vi "Main v0.97.vi"() -> ()   [LabVIEW 2017]
doc: "v0.85:\n- Counts for rejects and total\n\nv0.5:\n\n- Added Reject to Manual Mode\n- Send reject pallet cluster during manual mode\n- Run continuous manual happens only when no error has occured"
uses:
  Controls/Main Tabs v0.1.ctl
  Controls/Auto.ctl
  RT/Controls/Auto Delays.ctl
  RT/Controls/Auto Times.ctl
  Controls/UI Data.ctl
  support/Controls/Auto Stats.ctl
  support/Message Queue/Enqueue Message (Single).vi
  GV/Maintenance GV.vi
  <vilib>/Utility/error.llb/Error Cluster From Error Code.vi
  <vilib>/ErrorRing/Error Ring.xnode
  support/Message Queue/Message Queue.lvlib
  support/User Event - Stop/User Event - Stop.lvlib
panel:
  out "Shutdown?":bool
  out "Boolean 8":bool
  out "Boolean 7":bool
  out "Boolean 6":bool
  out "Boolean 5":bool
  out "Boolean 4":bool
  out "Boolean 3":bool
  out "Boolean 2":bool
  out "Boolean":bool
  in  "Reject Pallets":T1
  out "Date-Time":string caption="Dip-Tube Assembly Automation (HMI) v0.9"
  out "Main Tab":T2
  in  "Autocycle":T3
  in  "Manual":bool
  in  "Parameters":bool
  in  "Maintenance":bool
  in  "BF Para":cluster{"Delay 1":u32, "Delay 2":u32}={"Delay 1"=1000, "Delay 2"=1000}
  in  "Reject Para":cluster{"Delay":u32}={"Delay"=400}
  in  "Meas. Para":T4={"Delay"=500.0, "Mean Length"=188.9, "Tolerance"=1.0}
  in  "PF Para":cluster{"Delay":u32, "Timeout":u32}={"Delay"=1000, "Timeout"=1000}
  in  "Tube Feeder Para":T5={"Delay"=400, "Delay 2"=250, "Max Attempts"=250}
  in  "Cutting Para":T6={"Delay"=400, "Delay 2"=250, "Delay 3"=250}
  in  "Agitator Para":cluster{"Delay":u32, "Timeout":u32}={"Delay"=400, "Timeout"=250}
  in  "Insertion Para":cluster{"Delay 1":u32, "Delay 2":u32}={"Delay 1"=1000, "Delay 2"=1000}
  in  "Save Para":bool
  in  "Home Para":bool
  out "OEE":dbl format="%#.1f"
  out "QUA":dbl=100.0 min=0.0 max=100.0 step=0.1
  in  "Ideal Time":dbl=2.0 min=0.0 max=100.0 step=0.1
  in  "AVL":dbl=100.0 min=0.0 max=100.0 step=0.1
  out "Rejects 2":u32
  in  "Reset MCount":bool
  in  "Enable BF?":bool
  in  "Enable Agitate?":bool
  in  "Enable Reject?":bool
  in  "Toggle Motor":bool
  in  "Continuous?":bool
  in  "Enable Measure?":bool
  in  "Enable Index?":bool
  in  "Enable PF?":bool
  in  "Auto Para":T7={"Agitator Delays"=[400, 250], "TF Delays"=[700, 800, 2], "Insertion Delays"=[100, 500], "Cutting Delays"=[300, 300, 100], "PF Delays"=[250, 30000], "Measur. Delays"=[500.0, 188.9, 1.0], "Reject Delays"=[500], "BF Delays"=[1000, 1000]}
  in  "Enable Cutting?":bool
  in  "Enable Insertion?":bool
  in  "Run Manual":bool
  in  "Enable TF?":bool
  in  "Home Manual":bool
  out "Status 2":T9
  out "Measurements":T10 {"Height 1" format="%#.2f"; "Height 2" format="%#.2f"; "Height 3" format="%#.2f"; "Height 4" format="%#.2f"}
  out "Output Count":u32 caption="Output\nCount"
  out "PRF":dbl=100.0 min=0.0 max=100.0 step=0.1
  out "Statuses":string[][](table)
  in  "All IO":bool
  in  "Stats":bool
  in  "Home AC":bool
  out "Status":string
  out "Count":u32 format="%06.0f"
  out "Cycle Time":dbl format="%0.2f"
  out "Rejects":u32 format="%06.0f"
  out "Output Chart":T11(graph)
  out "Reject Count":u32
  out "Total Count":u32
  out "Total Time":dbl caption="Total Effective Cycle Time (s)" format="%#.3f"
  out "Time Chart":T12(graph)
  out "OEE Chart":cluster{"1":dbl, "2":dbl, "3":dbl, "4":dbl}(graph)
  out "Measurement Chart":cluster{"1":dbl, "2":dbl, "3":dbl, "4":dbl}(graph)
  out "Timestamp":string caption="Date & Timestamp"
  out "Latest Measure.":T13 caption="Latest Measurements" {"Length 1 (mm)" format="%#.2f"}
  out "Auto Times":T8
  in  "Back Stats":bool
  out "OEE 2":T14 caption="Latest Measurements" {"AVL" format="%#.1f"; "PRF" format="%#.1f"; "QUA" format="%#.1f"; "OEE" format="%#.1f"}
  out "IAS 4":dbl format="%#.3f"
  out "IAS 3":dbl format="%#.3f"
  out "IAS 2":dbl format="%#.3f"
  out "IAS 1":dbl format="%#.3f"
  out "DI 1":T15
  out "DI 2":T16
  out "DO 1":T17
  in  "Back IO":bool
  in  "Exit":bool
  in  "Shutdown":bool
  # "HARMONY VISION DIP-TUBE ASSEMBLY AUTOMATION"
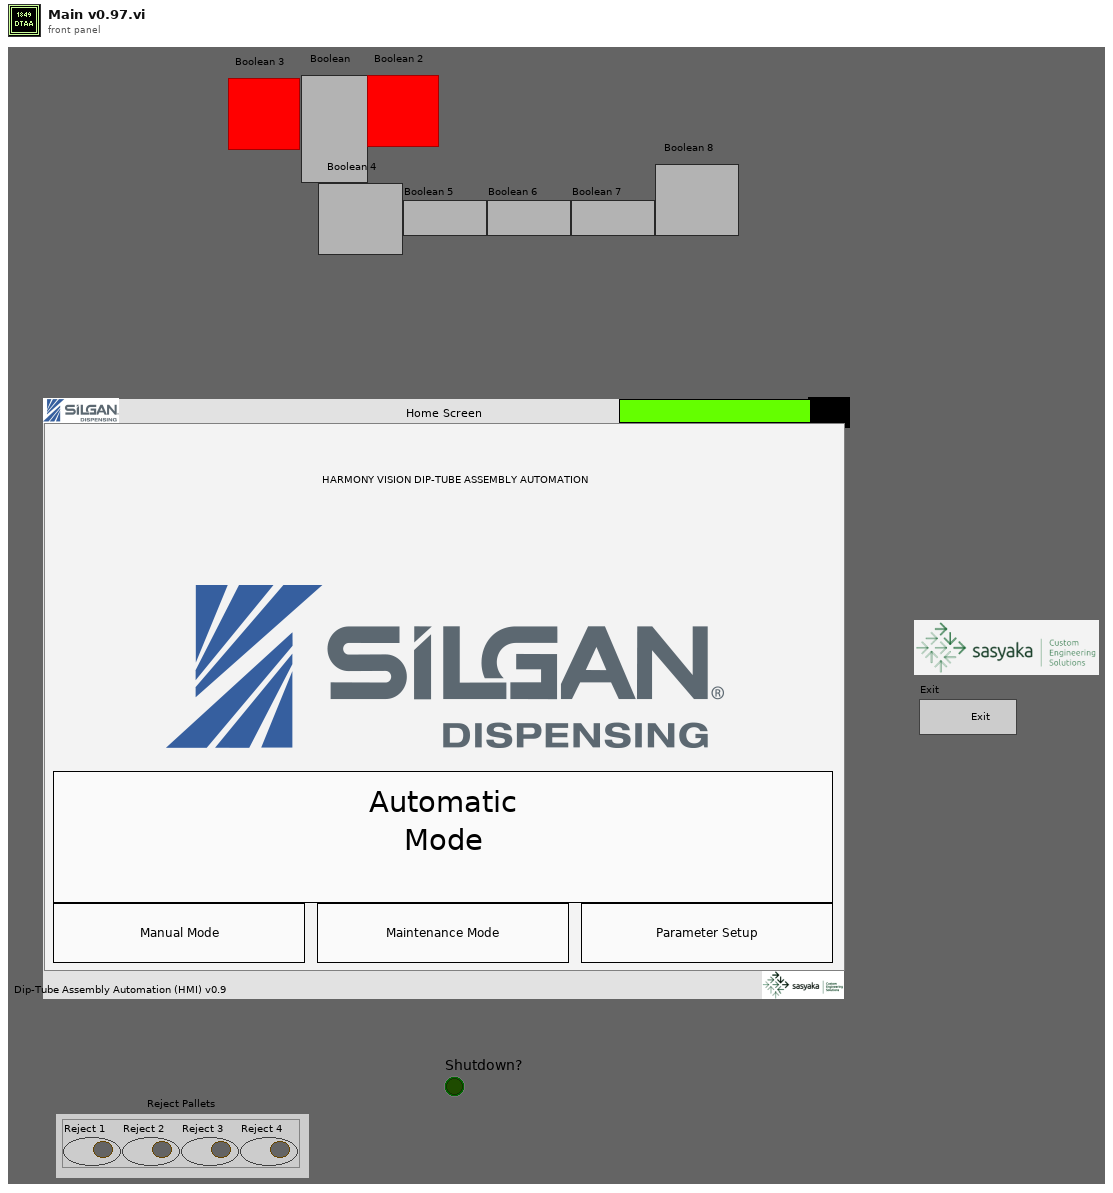
[diagram p1: front panel]
types:
  T1 = cluster{"Reject 1":bool, "Reject 2":bool, "Reject 3":bool, "Reject 4":bool}
  T2 = typedef "Main Tabs v0.1.ctl" = enum32{"Home Screen", "Parameter Setup", "Manual Mode", "Autocycle", "Autocycle Statistics", "Autocycle IOs"}
  T3 = typedef "Auto.ctl" = bool
  T4 = cluster{"Delay":dbl, "Mean Length":dbl, "Tolerance":dbl}
  T5 = cluster{"Delay":u32, "Delay 2":u32, "Max Attempts":u32}
  T6 = cluster{"Delay":u32, "Delay 2":u32, "Delay 3":u32}
  T7 = typedef "Auto Delays.ctl" = cluster{"Agitator Delays":u32[], "TF Delays":u32[], "Insertion Delays":u32[], "Cutting Delays":u32[], "PF Delays":u32[], "Measur. Delays":dbl[], "Reject Delays":u32[], "BF Delays":u32[]}
  T8 = typedef "Auto Times.ctl" = cluster{"Index Time":u32, "TF Time":u32, "Insertion Time":u32, "Cutting Time":u32, "PF Time":u32, "Meas. Time":u32, "Reject Time":u32}
  T9 = cluster{"Auto Times":T8, "error out":errorcluster}
  T10 = cluster{"Height 1":dbl, "Height 2":dbl, "Height 3":dbl, "Height 4":dbl}
  T11 = cluster{"OutputCount":u32, "Numeric Control":u32}
  T12 = cluster{"Index":dbl, "TF":dbl, "Insert":dbl, "Cutting":dbl, "PF":dbl, "Measure.":dbl, "Reject":dbl}
  T13 = cluster{"Length 1 (mm)":dbl, "Pallet 2 (mm)":dbl, "Pallet 3 (mm)":dbl, "Pallet 4 (mm)":dbl}
  T14 = cluster{"AVL":dbl, "PRF":dbl, "QUA":dbl, "OEE":dbl}
  T15 = cluster{"Machine_ON":bool, "E_stop ":bool, "SW_Pressure":bool, "SW_Start ":bool, "SW_Reset":bool, "SW_Stop":bool, "SW_Door":bool, "RS_Index_Rotary_CW":bool, "RS_Index_Rotary_CCW":bool, "RS_Index_Stopper _Rear":bool, "RS_Index_Output_Separator_Rear":bool, "PES_Index_Pallet_Sensor":bool, "PES_Index_Output_Part Sensor":bool, "ICS_BF_Low_Level_1":bool, "ICS_BF_Low_Level_2":bool, "ICS_BF_Pump_CNVR_Full_1":bool, "ICS_BF_Pump_CNVR_Full_2":bool, "ICS_BF_Pump_CNVR_Full_3":bool, "ICS_BF_Pump_CNVR_Full_4":bool, "PES_PC_Pump Presence_1":bool, "PES_PC_Pump Presence_2":bool, "PES_PC_Pump Presence_3":bool, "PES_PC_Pump Presence_4":bool, "RS_PC_Gating_Front":bool, "PES_Pump_Interference":bool, "PES_TF_Low_Level":bool, "PES_Tube Presence_1":bool, "PES_Tube Presence_2":bool, "PES_Tube Presence_3":bool, "PES_Tube Presence_4":bool, "DI1.30":bool, "DI1.31":bool}
  T16 = cluster{"RS_Agitatator_1_Rear ":bool, "RS_Agitatator_2_Rear ":bool, "RS_TF_Gating CYL_Rear":bool, "RS_Insertion_1_Rear":bool, "RS_Insertion_1_Front":bool, "RS_Insertion _2_Rear":bool, "RS_Insertion _2_Front":bool, "RS_Insertion _3_Rear":bool, "RS_Insertion _3_Front":bool, "RS_Insertion _4_Rear":bool, "RS_Insertion _4_Front":bool, "RS_Insertion_Clamp_Rear":bool, "RS_Cutting_Rear":bool, "RS_Cutting_Clamp _Rear":bool, "RS_Measurement_1_Rear":bool, "RS_Measurement_2_Rear":bool, "RS_Measurement_3_Rear":bool, "RS_Measurement_4_Rear":bool, "DI2.18":bool, "RS_Rejection_1_Rear":bool, "RS_Rejection_2_Rear":bool, "RS_Rejection_3_Rear":bool, "RS_Rejection_4_Rear":bool, "DI2.23":bool, "DI2.24":bool, "DI2.25":bool, "DI2.26":bool, "DI2.27":bool, "DI2.28":bool, "DI2.29":bool, "DI2.30":bool, "DI2.31":bool}
  T17 = cluster{"TL_Red":bool, "TL_Orange":bool, "TL_Green":bool, "TL_Buzzer":bool, "SOL_Index_Rotary_CW":bool, "SOL_Index_Rotary_CCW":bool, "SOL_Index_Stopper_Rear":bool, "SOL_OutputSeparator_Rear":bool, "Bowl  Feeder_ ON 1":bool, "Pump_CNVR_Motor _ON":bool, "SOL_PC_Gating_CYL_Rear":bool, "SOL_Tube_Feed_Agitatator":bool, "SOL_Tube_Feed_Gating_CYL":bool, "SOL_Insertion _CYL":bool, "SOL_Insertion_Clamp_CYL":bool, "SOL_Cutting_CYL":bool, "SOL_Cutting_Clamp_CYL":bool, "SOL_Insertion_Air_Nozzle":bool, "SOL_Measurement_CYL":bool, "DO1.19":bool, "SOL_Rejection CYL_1":bool, "SOL_Rejection CYL_2":bool, "SOL_Rejection CYL_3":bool, "SOL_Rejection CYL_4":bool, "Bowl  Feeder_ ON 2":bool, "SOL_BF_BlowerON":bool, "SOL_BF1_Track1":bool, "SOL_BF1_Track2":bool, "SOL_BF2_Track1":bool, "SOL_BF2_Track2":bool, "DO1.30":bool, "DO1.31":bool}
  T18 = typedef "UI Data.ctl" = cluster{"Main Tab":refnum<vi>}
  T19 = typedef "Message Queue.lvlib/All Message Queues.ctl" = cluster{"UI":refnum<queue>}
  T20 = enum8{"Enabled", "Disabled", "Disabled and Grayed Out"}
  T21 = cluster{"Array":string[][], "Machine Status":string}
  T22 = typedef "Auto Stats.ctl" = cluster{"Time":timestamp, "OEE":cluster{"AVL":dbl, "PRF":dbl, "QUA":dbl, "OEE":dbl}, "Auto Times":T8, "Counts out":cluster{"OutputCount":u32, "RejectCount":u32}, "Measurements":cluster{"1":dbl, "2":dbl, "3":dbl, "4":dbl}, "Outputs":cluster{"OutputCount":u32, "Numeric Control":u32}}
  T23 = cluster{"Auto Times":T8, "Results":cluster{"Measurements":cluster{"1":dbl, "2":dbl, "3":dbl, "4":dbl}, "Reject Pallets":cluster{"Reject 1":bool, "Reject 2":bool, "Reject 3":bool, "Reject 4":bool}}, "OutputCount":u32, "error out":errorcluster}
  T24 = enum8{"Information", "Error", "Successful", "Tips"}
  T25 = cluster{"Agitator Delays[0]":u32, "Agitator Delays[1]":u32}
  T26 = cluster{"TF Delays[0]":u32, "TF Delays[1]":u32, "TF Delays[2]":u32}
  T27 = cluster{"Insertion Delays[0]":u32, "Insertion Delays[1]":u32}
  T28 = cluster{"Cutting Delays[0]":u32, "Cutting Delays[1]":u32, "Cutting Delays[2]":u32}
  T29 = cluster{"Measur. Delays[0]":dbl, "Measur. Delays[1]":dbl, "Measur. Delays[2]":dbl}
  T30 = typedef "All Inputs.ctl" = cluster{"DI 1":cluster{"Machine_ON":bool, "E_stop ":bool, "SW_Pressure":bool, "SW_Start ":bool, "SW_Reset":bool, "SW_Stop":bool, "SW_Door":bool, "RS_Index_Rotary_CW":bool, "RS_Index_Rotary_CCW":bool, "RS_Index_Stopper _Rear":bool, "RS_Index_Output_Separator_Rear":bool, "PES_Index_Pallet_Sensor":bool, "PES_Index_Output_Part Sensor":bool, "ICS_BF_Low_Level_1":bool, "ICS_BF_Low_Level_2":bool, "ICS_BF_Pump_CNVR_Full_1":bool, "ICS_BF_Pump_CNVR_Full_2":bool, "ICS_BF_Pump_CNVR_Full_3":bool, "ICS_BF_Pump_CNVR_Full_4":bool, "PES_PC_Pump Presence_1":bool, "PES_PC_Pump Presence_2":bool, "PES_PC_Pump Presence_3":bool, "PES_PC_Pump Presence_4":bool, "RS_PC_Gating_Front":bool, "PES_Pump_Interference":bool, "PES_TF_Low_Level":bool, "PES_Tube Presence_1":bool, "PES_Tube Presence_2":bool, "PES_Tube Presence_3":bool, "PES_Tube Presence_4":bool, "DI1.30":bool, "DI1.31":bool}, "DI 2":cluster{"RS_Agitatator_1_Rear ":bool, "RS_Agitatator_2_Rear ":bool, "RS_TF_Gating CYL_Rear":bool, "RS_Insertion_1_Rear":bool, "RS_Insertion_1_Front":bool, "RS_Insertion _2_Rear":bool, "RS_Insertion _2_Front":bool, "RS_Insertion _3_Rear":bool, "RS_Insertion _3_Front":bool, "RS_Insertion _4_Rear":bool, "RS_Insertion _4_Front":bool, "RS_Insertion_Clamp_Rear":bool, "RS_Cutting_Rear":bool, "RS_Cutting_Clamp _Rear":bool, "RS_Measurement_1_Rear":bool, "RS_Measurement_2_Rear":bool, "RS_Measurement_3_Rear":bool, "RS_Measurement_4_Rear":bool, "RS_Measure_Clamp_Rear":bool, "RS_Rejection_1_Rear":bool, "RS_Rejection_2_Rear":bool, "RS_Rejection_3_Rear":bool, "RS_Rejection_4_Rear":bool, "DI2.23":bool, "DI2.24":bool, "DI2.25":bool, "DI2.26":bool, "DI2.27":bool, "DI2.28":bool, "DI2.29":bool, "DI2.30":bool, "DI2.31":bool}, "IAS 1":dbl, "IAS 2":dbl, "IAS 3":dbl, "IAS 4":dbl, "DO 1":cluster{"TL_Red":bool, "TL_Orange":bool, "TL_Green":bool, "TL_Buzzer":bool, "SOL_Index_Rotary_CW":bool, "SOL_Index_CNVR_Rotary_CCW":bool, "SOL_Index_CNVR_Stopper_Rear":bool, "SOL_Index_CNVR_Output _Separator _Rear":bool, "Bowl  Feeder_ ON 1":bool, "Pump_CNVR_Motor _ON":bool, "SOL_PC_Gating_CYL_Rear":bool, "SOL_Tube_Feed_Agitatator":bool, "SOL_Tube_Feed_Gating_CYL":bool, "SOL_Insertion _CYL":bool, "SOL_Insertion_Clamp_CYL":bool, "SOL_Cutting_CYL":bool, "SOL_Cutting_Clamp_CYL":bool, "SOL_Insertion_Air_Nozzle":bool, "SOL_Measurement_CYL":bool, "DO1.19":bool, "SOL_Rejection CYL_1":bool, "SOL_Rejection CYL_2":bool, "SOL_Rejection CYL_3":bool, "SOL_Rejection CYL_4":bool, "Bowl  Feeder_ ON 2":bool, "SOL_BF_BlowerON":bool, "SOL_BF1_Track1":bool, "SOL_BF1_Track2":bool, "SOL_BF2_Track1":bool, "SOL_BF2_Track2":bool, "DO1.30":bool, "DO1.31":bool}}
  T31 = cluster{"RS_Agitatator_1_Rear ":bool, "RS_Agitatator_2_Rear ":bool, "RS_TF_Gating CYL_Rear":bool, "RS_Insertion_1_Rear":bool, "RS_Insertion_1_Front":bool, "RS_Insertion _2_Rear":bool, "RS_Insertion _2_Front":bool, "RS_Insertion _3_Rear":bool, "RS_Insertion _3_Front":bool, "RS_Insertion _4_Rear":bool, "RS_Insertion _4_Front":bool, "RS_Insertion_Clamp_Rear":bool, "RS_Cutting_Rear":bool, "RS_Cutting_Clamp _Rear":bool, "RS_Measurement_1_Rear":bool, "RS_Measurement_2_Rear":bool, "RS_Measurement_3_Rear":bool, "RS_Measurement_4_Rear":bool, "RS_Measure_Clamp_Rear":bool, "RS_Rejection_1_Rear":bool, "RS_Rejection_2_Rear":bool, "RS_Rejection_3_Rear":bool, "RS_Rejection_4_Rear":bool, "DI2.23":bool, "DI2.24":bool, "DI2.25":bool, "DI2.26":bool, "DI2.27":bool, "DI2.28":bool, "DI2.29":bool, "DI2.30":bool, "DI2.31":bool}
  T32 = cluster{"TL_Red":bool, "TL_Orange":bool, "TL_Green":bool, "TL_Buzzer":bool, "SOL_Index_Rotary_CW":bool, "SOL_Index_CNVR_Rotary_CCW":bool, "SOL_Index_CNVR_Stopper_Rear":bool, "SOL_Index_CNVR_Output _Separator _Rear":bool, "Bowl  Feeder_ ON 1":bool, "Pump_CNVR_Motor _ON":bool, "SOL_PC_Gating_CYL_Rear":bool, "SOL_Tube_Feed_Agitatator":bool, "SOL_Tube_Feed_Gating_CYL":bool, "SOL_Insertion _CYL":bool, "SOL_Insertion_Clamp_CYL":bool, "SOL_Cutting_CYL":bool, "SOL_Cutting_Clamp_CYL":bool, "SOL_Insertion_Air_Nozzle":bool, "SOL_Measurement_CYL":bool, "DO1.19":bool, "SOL_Rejection CYL_1":bool, "SOL_Rejection CYL_2":bool, "SOL_Rejection CYL_3":bool, "SOL_Rejection CYL_4":bool, "Bowl  Feeder_ ON 2":bool, "SOL_BF_BlowerON":bool, "SOL_BF1_Track1":bool, "SOL_BF1_Track2":bool, "SOL_BF2_Track1":bool, "SOL_BF2_Track2":bool, "DO1.30":bool, "DO1.31":bool}
  T33 = cluster{"Auto Para":T7, "Reject Pallets":cluster{"Reject 1":bool, "Reject 2":bool, "Reject 3":bool, "Reject 4":bool}}
  T34 = cluster{"Measurements":cluster{"1":dbl, "2":dbl, "3":dbl, "4":dbl}, "Reject Pallets":cluster{"Reject 1":bool, "Reject 2":bool, "Reject 3":bool, "Reject 4":bool}}
  T35 = cluster{"Reject Pallets":cluster{"Reject 1":bool, "Reject 2":bool, "Reject 3":bool, "Reject 4":bool}, "Measurements":cluster{"1":dbl, "2":dbl, "3":dbl, "4":dbl}}
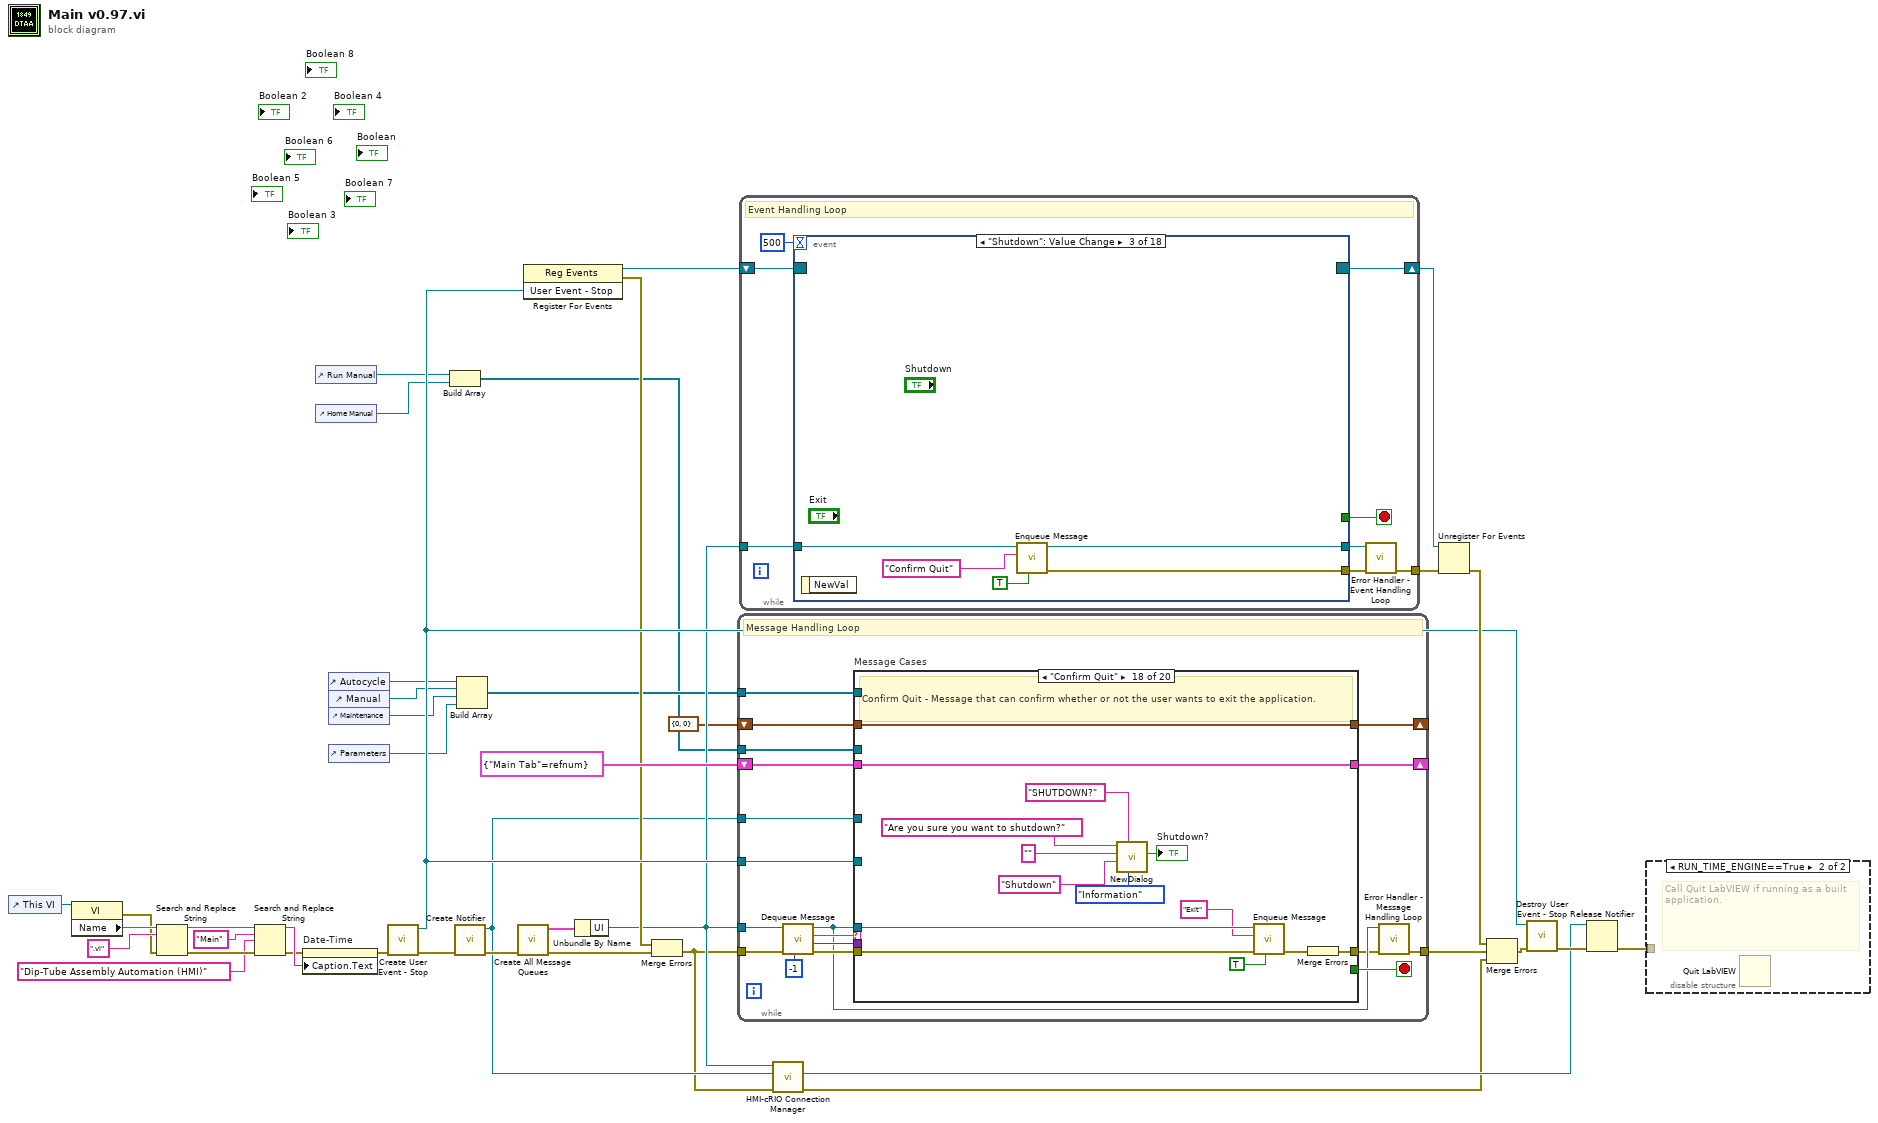
[diagram p0: block diagram]
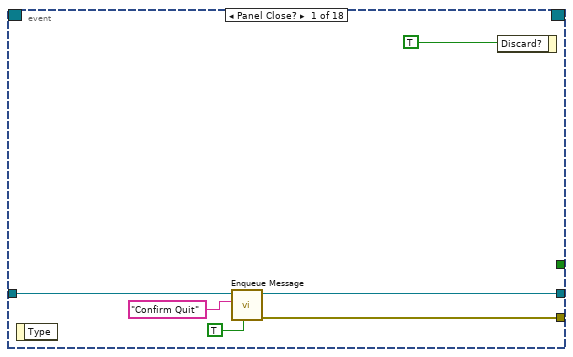
[diagram p2: hidden frame]
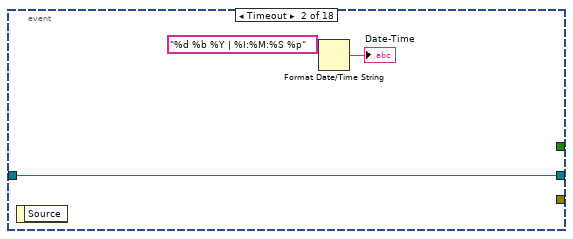
[diagram p3: hidden frame]
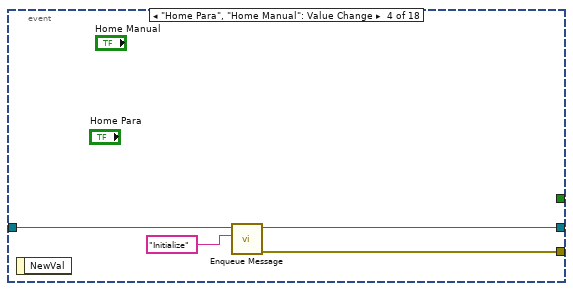
[diagram p4: hidden frame]
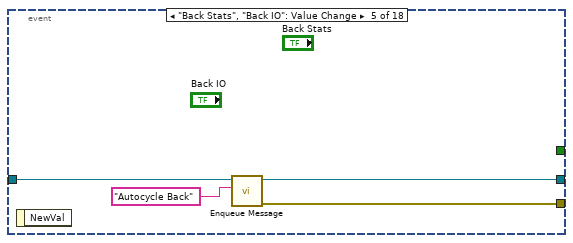
[diagram p5: hidden frame]
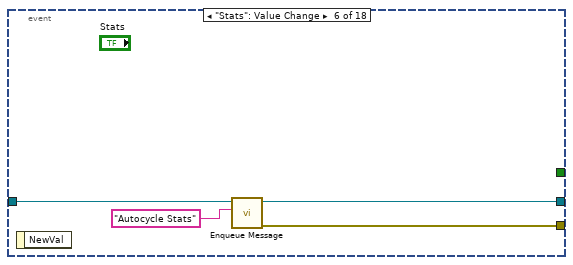
[diagram p6: hidden frame]
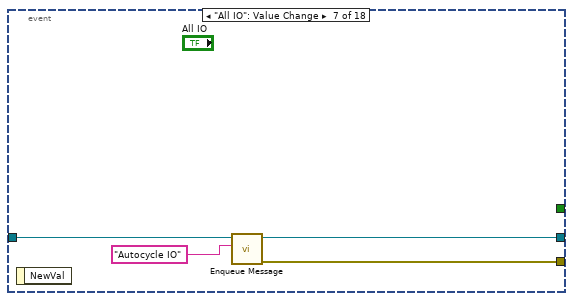
[diagram p7: hidden frame]
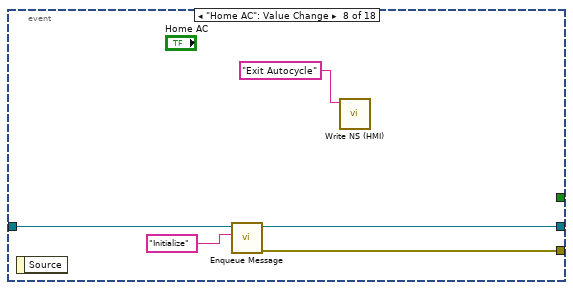
[diagram p8: hidden frame]
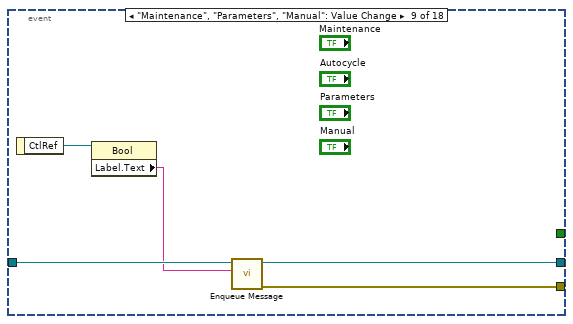
[diagram p9: hidden frame]
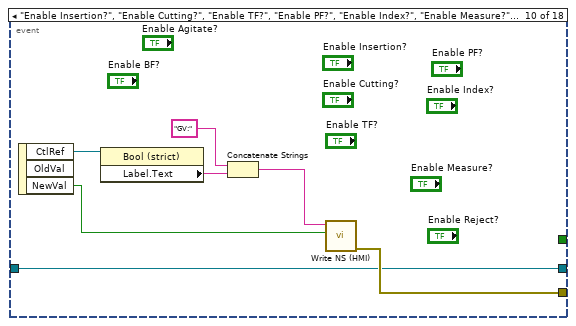
[diagram p10: hidden frame]
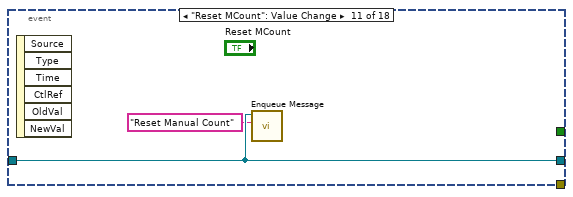
[diagram p11: hidden frame]
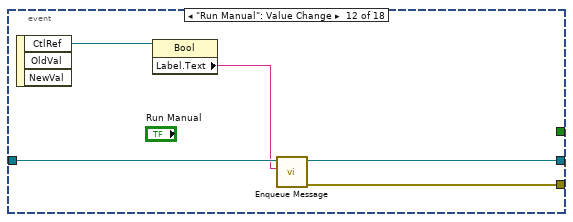
[diagram p12: hidden frame]
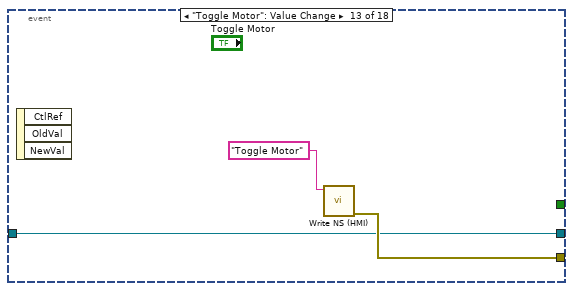
[diagram p13: hidden frame]
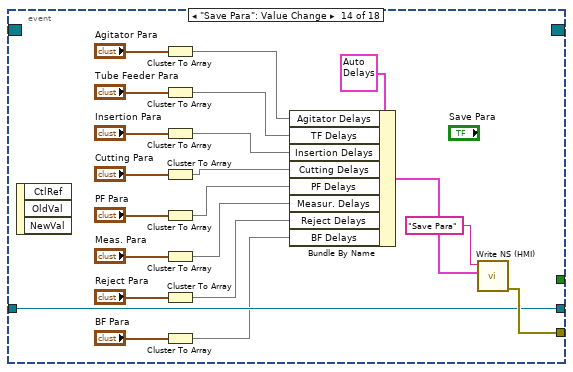
[diagram p14: hidden frame]
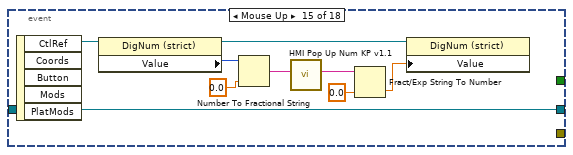
[diagram p15: hidden frame]
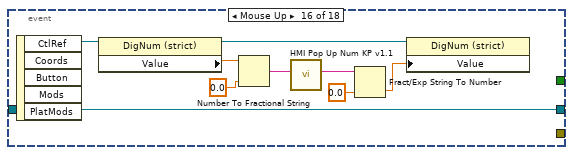
[diagram p16: hidden frame]
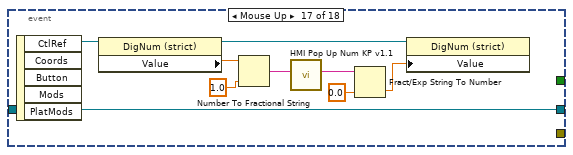
[diagram p17: hidden frame]
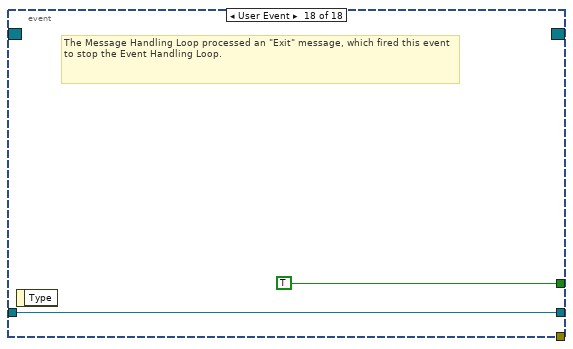
[diagram p18: hidden frame]
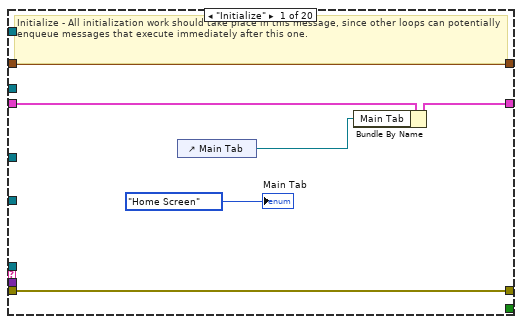
[diagram p19: hidden frame]
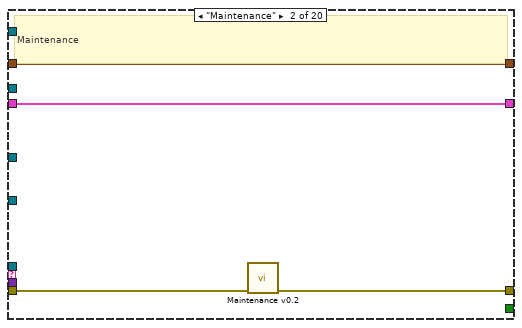
[diagram p20: hidden frame]
diagram:
  n1 = control-ref of="This VI"() -> (w11:refnum<vi>)
  n2 = property class="VI"(reference=w11) -> (error out=w10:errorcluster, "Name"=w17:string)  [unwired: 1 in, 1 out]
  n3 = Search and Replace String(input string=w17, search string=".vi", error in=w10) -> (result string=w15:string, error out=w14:errorcluster)  [unwired: 5 in, 2 out]
  n4 = Search and Replace String(input string=w15, search string="Main", replace string="Dip-Tube Assembly Automation (HMI)" ("replace string (\"\")"), error in=w14) -> (result string=w9:string, error out=w8:errorcluster)  [unwired: 4 in, 2 out]
  n5 = property on="Date-Time" class="Str"(error in=w8, "Caption.Text"=w9) -> (error out=w7:errorcluster)  [unwired: 1 in, 1 out]
  n6 = control-ref of="Run Manual"() -> (w6:refnum<vi>)
  n7 = control-ref of="Home Manual"() -> (w5:refnum<vi>)
  n8 = control-ref of="Autocycle"() -> (w22:refnum<vi>)
  n9 = control-ref of="Manual"() -> (w21:refnum<vi>)
  n10 = control-ref of="Maintenance"() -> (w20:refnum<vi>)
  n11 = control-ref of="Parameters"() -> (w19:refnum<vi>)
  n12 = call "Create User Event - Stop.vi"("error in (no error)"=w7) -> ("error out"=w28:errorcluster, "User Event - Stop"=w31:refnum<user-event>)  [unwired: 9 in]
  n13 = Build Array(w6, w5) -> (w4:refnum<vi>[])
  n14 = call "Create Notifier.vi"("error in (no error)"=w28) -> ("error out"=w27:errorcluster, "notifier out"=w2:refnum<notifier>)  [unwired: 9 in]
  n15 = Build Array(w22, w21, w20, w19) -> (w18:refnum<vi>[])
  n16 = call "Create All Message Queues.vi"("error in (no error)"=w27) -> ("error out"=w40:errorcluster, "Message Queues out"=w39:T19)  [unwired: 9 in]
  n17 = register-events(w31) -> (reference out=w32:refnum<event-registration>, error out=w30:errorcluster)  [unwired: 2 in]
  n18 = Unbundle By Name(w39) -> ("UI"=w29:refnum<queue>)
  n19 = Merge Errors(w30, w40) -> (w1:errorcluster)
  n20 = while {
    tunnel: w29 -> [w51]
    shift-right: [w58] -> _
    shift-left: T18 {"Main Tab"=refnum} ("Data Cluster") -> [w41]
    tunnel: w31 -> [w56]
    tunnel: w1 -> [w55]
    tunnel: [w49] -> w38
    tunnel: w2 -> [w46]
    tunnel: w18 -> [w45]
    tunnel: w4 -> [w44]
    shift-right: [w42] -> _
    shift-left: cluster{"OutputCount":u32, "RejectCount":u32} {"OutputCount"=0, "RejectCount"=0} -> [w43]
    stop <- w57 stop-if-true
    # "Message Handling Loop"
    n21 = call "Dequeue Message.vi"("timeout"=-1, "error in (no error)"=w55, "Message Queue"=w51) -> ("error out"=w54:errorcluster, "Message Data"=w52:variant, "Message"=w53:string, "dup Message Queue"=w50:refnum<queue>)  [unwired: 5 in]
    n22 = case "Message Cases" shown="\"Confirm Quit\"" w53 {
      selector: w53 -> [_ _ _ _ _ _ _ _ _ _ _ _ _ _ _ _ _ _ _ w317]
      tunnel: w50 -> [_ _ _ _ _ _ _ _ _ w154 w162 _ _ _ w245 _ _ w296 w315 _]
      tunnel: w54 -> [w64 w67 w80 w86 w112 w127 w134 w144 w149 w156 w170 w192 w211 w221 w253 w263 w286 w300 w308 _]
      tunnel: [w64 w66 w79 w85 w111 w127 w133 w144 w149 w155 w169 w193 w212 w223 w244 w263 w281 w298 w311 w318] -> w48
      tunnel: w41 -> [w63 w68 w82 w91 w114 w126 w130 w148 w153 w161 w167 w194 w213 w224 w254 w262 w285 w299 w314 w319]
      tunnel: [w62 w68 w82 w91 w114 w126 w130 w148 w153 w161 w167 w194 w213 w224 w254 w262 w285 w299 w314 w319] -> w58
      tunnel: [_ _ _ _ _ _ _ _ _ _ _ _ _ _ _ _ _ _ TRUE _] -> w57
      tunnel: w52 -> [_ _ w78 _ w110 _ _ _ _ _ _ w191 w210 _ w252 _ w284 _ w305 _]
      tunnel: w56 -> [_ _ _ _ _ _ _ _ _ _ _ _ _ _ _ _ _ _ w310 _]
      tunnel: w46 -> [_ _ _ _ _ _ _ _ _ _ _ _ _ _ _ _ _ _ w304 _]
      tunnel: w45 -> [_ _ w74 _ _ _ _ _ _ _ _ _ _ _ _ _ _ _ _ _]
      tunnel: w44 -> [_ _ _ _ _ _ _ _ _ _ _ _ _ w218 w250 _ _ _ _ _]
      tunnel: w43 -> [w59 w65 w69 w88 w113 w115 w135 w145 w150 w158 w171 w189 w208 w214 w243 _ w280 w293 w301 w316]
      tunnel: [w59 w65 w69 w88 w113 w115 w135 w145 w150 w158 w171 w189 w208 w214 w238 cluster{"OutputCount":u32, "RejectCount":u32} {"OutputCount"=0, "RejectCount"=0} w280 w293 w301 w316] -> w42
      frame "Initialize" {
        # "Initialize - All initialization work should take place in this message, since other loops can potentially enqueue messages that execute immediately after this one."
        n23 = control-ref of="Main Tab"() -> (w61:refnum<vi>)
        n24 = Bundle By Name(cluster=w63, "Main Tab"=w61) -> (w62:T18)
        "Main Tab" <- Main_Tabs_v0.1."Home Screen" ("Main Tab")
      }
      frame "Maintenance" {
        # "Maintenance"
        n25 = call "Maintenance v0.2.vi"("Error In"=w67) -> ("Error out"=w66:errorcluster)  [unwired: 10 in]
      }
      frame "Connection" {
        n26 = Variant To Data(error in=w80, type=FALSE, Variant=w78) -> (data=w73:bool, error out=w79:errorcluster)
        n27 = Select(t=u32 6618880 ("Text.Text Colors:BG Color"), s=w73, f=u32 16762112 ("Text.Text Colors:BG Color")) -> (s? t:f=w75:u32)
        n28 = property on="Date-Time" class="Str"("Text.BGColor"=w75) -> ()  [unwired: 2 in, 2 out]
        n29 = Select(t=T20."Enabled" ("Disabled"), s=w73, f=T20."Disabled and Grayed Out") -> (s? t:f=w71:T20)
        n30 = for {
          tunnel: w74 -> [w84] mode=indexing
          tunnel: w71 -> [w83]
          n31 = property class="Bool"(reference=w84, "DisabledEnum"=w83) -> ()  [unwired: 1 in, 2 out]
        }
      }
      frame "Parameters" {
        # "Parameters"
        n32 = Unbundle By Name(w91) -> ("Main Tab"=w90:refnum<vi>)
        n33 = call "Write NS (HMI).vi"("error in (no error)"=w86, "Message"="Enter Para") -> ("error out"=w85:errorcluster)  [unwired: 9 in]
        n34 = property class="TabCtl"(reference=w90, "Value"=Main_Tabs_v0.1."Parameter Setup" ("Main Tab")) -> ()  [unwired: 1 in, 2 out]
      }
      frame "Current Para" {
        # "Parameters"
        n35 = Variant To Data(error in=w112, type=T7 {"Agitator Delays"=[1000], "TF Delays"=[1000], "Insertion Delays"=[1000], "Cutting Delays"=[1000], "PF Delays"=[1000], "Measur. Delays"=[1000.0], "Reject Delays"=[1000], "BF Delays"=[1000]} ("Auto Para"), Variant=w110) -> (data=w108:T7, error out=w111:errorcluster)
        n36 = Unbundle(w108) -> ("Agitator Delays"=w107:u32[], "TF Delays"=w106:u32[], "Insertion Delays"=w105:u32[], "Cutting Delays"=w104:u32[], "PF Delays"=w103:u32[], "Measur. Delays"=w102:dbl[], "Reject Delays"=w101:u32[], "BF Delays"=w100:u32[])
        n37 = property on="Auto Para" class="Clust (strict)"("Value"=w108) -> ()  [unwired: 2 in, 2 out]
        n38 = Array To Cluster(array=w107) -> (cluster=w99:T25)
        n39 = Array To Cluster(array=w106) -> (cluster=w98:T26)
        n40 = Array To Cluster(array=w105) -> (cluster=w97:T27)
        n41 = Array To Cluster(array=w104) -> (cluster=w96:T28)
        n42 = Array To Cluster(array=w103) -> (cluster=w95:cluster{"PF Delays[0]":u32, "PF Delays[1]":u32})
        n43 = Array To Cluster(array=w102) -> (cluster=w94:T29)
        n44 = Array To Cluster(array=w101) -> (cluster=w93:cluster{"Reject Delays[0]":u32})
        n45 = Array To Cluster(array=w100) -> (cluster=w92:cluster{"BF Delays[0]":u32, "BF Delays[1]":u32})
        n46 = property on="Agitator Para" class="Clust (strict)"("Value"=w99) -> ()  [unwired: 2 in, 2 out]
        n47 = property on="Tube Feeder Para" class="Clust (strict)"("Value"=w98) -> ()  [unwired: 2 in, 2 out]
        n48 = property on="Insertion Para" class="Clust (strict)"("Value"=w97) -> ()  [unwired: 2 in, 2 out]
        n49 = property on="Cutting Para" class="Clust (strict)"("Value"=w96) -> ()  [unwired: 2 in, 2 out]
        n50 = property on="PF Para" class="Clust (strict)"("Value"=w95) -> ()  [unwired: 2 in, 2 out]
        n51 = property on="Meas. Para" class="Clust (strict)"("Value"=w94) -> ()  [unwired: 2 in, 2 out]
        n52 = property on="Reject Para" class="Clust (strict)"("Value"=w93) -> ()  [unwired: 2 in, 2 out]
        n53 = property on="BF Para" class="Clust (strict)"("Value"=w92) -> ()  [unwired: 2 in, 2 out]
      }
      frame "Manual" {
        # "Parameters"
        n54 = control-ref of="Enable Index?"() -> (w123:refnum<vi>)
        n55 = control-ref of="Enable PF?"() -> (w122:refnum<vi>)
        n56 = control-ref of="Enable Cutting?"() -> (w121:refnum<vi>)
        n57 = control-ref of="Enable Insertion?"() -> (w120:refnum<vi>)
        n58 = control-ref of="Enable TF?"() -> (w119:refnum<vi>)
        n59 = control-ref of="Enable Measure?"() -> (w117:refnum<vi>)
        n60 = control-ref of="Enable Reject?"() -> (w116:refnum<vi>)
        n61 = Build Array(w123, w122, w121, w120, w119, w117, w116) -> (w118:refnum<vi>[])
        n62 = for {
          tunnel: w118 -> [w129] mode=indexing
          n63 = property class="Bool (strict)"(reference=w129, "Val(Sgnl)"=FALSE ("Value (Signaling)")) -> ()  [unwired: 1 in, 2 out]
        }
        n64 = Unbundle By Name(w126) -> ("Main Tab"=w125:refnum<vi>)
        n65 = property class="TabCtl"(reference=w125, "Value"=Main_Tabs_v0.1."Manual Mode" ("Main Tab")) -> ()  [unwired: 1 in, 2 out]
      }
      frame "Autocycle" {
        # "Parameters"
        n66 = call "Select Model.vi"() -> ("Cancel out"=w131:bool, "Model out"=w132:string)  [unwired: 10 in]
        n67 = case shown="False" w131 {
          tunnel: w134 -> [w141 w143]
          tunnel: [w140 w143] -> w133
          tunnel: w132 -> [w139 _]
          tunnel: w130 -> [w136 _]
          frame False {
            n68 = Unbundle By Name(w136) -> ("Main Tab"=w138:refnum<vi>)
            n69 = call "Write NS (HMI).vi"("error in (no error)"=w141, "Message Data"=w139, "Message"="Autocycle") -> ("error out"=w140:errorcluster)  [unwired: 8 in]
            n70 = property class="TabCtl"(reference=w138, "Value"=Main_Tabs_v0.1."Autocycle" ("Main Tab")) -> ()  [unwired: 1 in, 2 out]
          }
          frame True {
          }
        }
      }
      frame "Autocycle Back" {
        # "Parameters"
        n71 = Unbundle By Name(w148) -> ("Main Tab"=w147:refnum<vi>)
        n72 = property class="TabCtl"(reference=w147, "Value"=Main_Tabs_v0.1."Autocycle" ("Main Tab")) -> ()  [unwired: 1 in, 2 out]
      }
      frame "Autocycle Stats" {
        # "Parameters"
        n73 = Unbundle By Name(w153) -> ("Main Tab"=w152:refnum<vi>)
        n74 = property class="TabCtl"(reference=w152, "Value"=Main_Tabs_v0.1."Autocycle Statistics" ("Main Tab")) -> ()  [unwired: 1 in, 2 out]
      }
      frame "Autocycle IO" {
        # "Parameters"
        n75 = Unbundle By Name(w161) -> ("Main Tab"=w160:refnum<vi>)
        n76 = property class="TabCtl"(reference=w160, "Value"=Main_Tabs_v0.1."Autocycle IOs" ("Main Tab")) -> ()  [unwired: 1 in, 2 out]
        n77 = call-poly "Enqueue Message.vi"("error in (no error)"=w156, "Message"="Update IO", "Message Queue"=w154) -> ("error out"=w155:errorcluster)  [unwired: 7 in, 1 out]
      }
      frame "Update IO" {
        n78 = Unbundle By Name(w167) -> ("Main Tab"=w168:refnum<vi>)
        n79 = Wait (ms)(milliseconds to wait=u32 200) -> ()  [unwired: 1 out]
        n80 = property class="TabCtl"(reference=w168) -> ("Value"=w166:variant)  [unwired: 1 in, 2 out]
        n81 = Variant To Data(type=Main_Tabs_v0.1."Autocycle IOs" ("Main Tab"), Variant=w166) -> (data=w163:T2)  [unwired: 1 in, 1 out]
        n82 = global read "Maintenance GV.vi" "All IO"() -> (w172:T30)
        n83 = case shown="\"Autocycle IOs\"" w163 {
          tunnel: w170 -> [w180 w183]
          tunnel: [w180 w182] -> w169
          tunnel: w162 -> [_ w181]
          frame Default {
          }
          frame "Autocycle IOs" {
            n84 = call-poly "Enqueue Message.vi"("error in (no error)"=w183, "Message"="Update IO", "Message Queue"=w181) -> ("error out"=w182:errorcluster)  [unwired: 7 in, 1 out]
          }
        }
        n85 = Unbundle(w172) -> ("DI 1"=→"DI 1":T15, "DI 2"=→"DI 2":T31, "IAS 1"=→"IAS 1":dbl, "IAS 2"=→"IAS 2":dbl, "IAS 3"=→"IAS 3":dbl, "IAS 4"=→"IAS 4":dbl, "DO 1"=→"DO 1":T32)
      }
      frame "Update UI" {
        # "Update Display - Convert the message data to a string to display in the Data Display indicator."
        n86 = Variant To Data(error in=w192, type=T21 {"Array"=[], "Machine Status"=""} ("Status Cluster"), Variant=w191) -> (data=w187:T21, error out=w190:errorcluster)
        n87 = Unbundle(w187) -> ("Array"=→"Statuses":string[][], "Machine Status"=→"Status":string)
        n88 = Merge Errors(w190) -> (w193:errorcluster)
      }
      frame "Autocycle Log" {
        # "Update Display - Convert the message data to a string to display in the Data Display indicator."
        n89 = Variant To Data(error in=w211, type=T22 {"Time"=timestamp(0 s since 1904-01-01), "OEE"={"AVL"=100.0, "PRF"=100.0, "QUA"=100.0, "OEE"=0.0}, "Auto Times"={"Index Time"=0, "TF Time"=0, "Insertion Time"=0, "Cutting Time"=0, "PF Time"=0, "Meas. Time"=0, "Reject Time"=0}, "Counts out"={"OutputCount"=0, "RejectCount"=0}, "Measurements"={"1"=0.0, "2"=0.0, "3"=0.0, "4"=0.0}, "Outputs"={"OutputCount"=0, "Numeric Control"=0}} ("Auto Stats"), Variant=w210) -> (data=w206:T22, error out=w209:errorcluster)
        n90 = call "Stats Unbundle.vi"("Auto Stats"=w206) -> ("Cycle Time"=→"Cycle Time" →"Total Time":dbl, "RejectCount"=→"Rejects" →"Reject Count":u32, "OutputCount"=→"Count" →"Total Count":u32, "Total Times"=→"Time Chart":T12)  [unwired: 7 in]
        n91 = Unbundle(w206) -> ("Time"=w204:timestamp, "OEE"=→"OEE Chart" →"OEE 2":T14, "Auto Times"=→"Auto Times":T8, "Measurements"=→"Latest Measure." →"Measurement Chart":cluster{"1":dbl, "2":dbl, "3":dbl, "4":dbl}, "Outputs"=→"Output Chart":T11)  [unwired: 1 out]
        n92 = Format Date/Time String(time format string (%c)="%d-%m-%Y | %H:%M:%S%3u", seconds (now)=w204) -> (date/time string=→"Timestamp":string)  [unwired: 1 in]
        n93 = Merge Errors(w209) -> (w212:errorcluster)
      }
      frame "Run Manual" {
        # "Update Manual mode"
        n94 = Bundle("Auto Para"="Auto Para", "Reject Pallets"="Reject Pallets") -> (w215:T33)  [unwired: 1 in]
        n95 = for {
          tunnel: w218 -> [w226] mode=indexing
          tunnel: T20."Disabled and Grayed Out" ("Disabled") -> [w225]
          n96 = property class="Bool"(reference=w226, "DisabledEnum"=w225) -> ()  [unwired: 1 in, 2 out]
        }
        n97 = call "Write NS (HMI).vi"("error in (no error)"=w221, "Message Data"=w215, "Message"="Manual Run") -> ("error out"=w220:errorcluster)  [unwired: 8 in]
        n98 = Merge Errors(w220) -> (w223:errorcluster)
      }
      frame "Manual Status" {
        n99 = Variant To Data(error in=w253, type=T23 {"Auto Times"={"Index Time"=0, "TF Time"=0, "Insertion Time"=0, "Cutting Time"=0, "PF Time"=0, "Meas. Time"=0, "Reject Time"=0}, "Results"={"Measurements"={"1"=0.0, "2"=0.0, "3"=0.0, "4"=0.0}, "Reject Pallets"={"Reject 1"=FALSE, "Reject 2"=FALSE, "Reject 3"=FALSE, "Reject 4"=FALSE}}, "OutputCount"=0, "error out"={"status"=FALSE, "code"=0, "source"=""}} ("cluster"), Variant=w252) -> (data=w249:T23, error out=w244:errorcluster)
        n100 = Unbundle(w249) -> ("Auto Times"=w248:T8, "Results"=w240:T34, "OutputCount"=w239:u32, "error out"=w242:errorcluster)
        n101 = for {
          tunnel: w250 -> [w259] mode=indexing
          tunnel: T20."Enabled" ("Disabled") -> [w258]
          n102 = property class="Bool"(reference=w259, "DisabledEnum"=w258) -> ()  [unwired: 1 in, 2 out]
        }
        n103 = Unbundle(w240) -> ("Measurements"=w228:cluster{"1":dbl, "2":dbl, "3":dbl, "4":dbl}, "Reject Pallets"=w229:T1)
        "Measurements" <- w228
        n104 = Bundle("Auto Times"=w248, "error out"=w242) -> (→"Status 2":T9)  [unwired: 1 in]
        n105 = Bundle("Reject Pallets"=w229, "Measurements"=w228) -> (w227:T35)  [unwired: 1 in]
        n106 = call "Counts Update (manual).vi"("output cluster"=w227, "Desired Cycle Time (s)"="Ideal Time", "AVL"="AVL", "OutputCount"=w239, "Counts in"=w243) -> ("OEE"=w233:T14, "Counts out"=w238:cluster{"OutputCount":u32, "RejectCount":u32})  [unwired: 4 in, 1 out]
        n107 = Unbundle(w233) -> ("PRF"=→"PRF":dbl, "QUA"=→"QUA":dbl, "OEE"=→"OEE":dbl)  [unwired: 1 out]
        n108 = Unbundle(w238) -> ("OutputCount"=→"Output Count":u32, "RejectCount"=→"Rejects 2":u32)
        n109 = case shown="True" "Continuous?" {
          tunnel: w245 -> [_ w257]
          tunnel: w242 -> [_ w256]
          frame False {
          }
          frame True {
            # "Run if continuous is TRUE & No Error"
            n110 = call-poly "Enqueue Message.vi"("error in (no error)"=w256, "Message"="Run Manual", "Message Queue"=w257) -> ()  [unwired: 7 in, 2 out]
          }
        }
      }
      frame "Reset Manual Count" {
        w260 = u32 0 ("Rejects")
        n111 = local write "Rejects 2"(w260) -> ()
        n112 = local write "Output Count"(w260) -> ()
      }
      frame "Error" {
        w267 = 128  # call and forget
        # "Run async so that this loop will continue to run"
        # "Error"
        n113 = Variant To Data(error in=w286, type=errorcluster {"status"=FALSE, "code"=0, "source"=""} ("error constant"), Variant=w284) -> (data=w279:errorcluster, error out=w282:errorcluster)
        n114 = Unbundle By Name(w279) -> ("source"=w278:string)
        n115 = vi-ref "NewDialog.vi"() -> (w274:refnum<vi>)
        n116 = property class="VI"(reference=w274) -> (error out=w276:errorcluster, "Name"=w275:string)  [unwired: 1 in, 1 out]
        n117 = Search and Replace String(input string=w278, search string="<err>") -> (result string=w266:string)  [unwired: 6 in, 3 out]
        n118 = Open VI Reference(type specifier VI Refnum (for type only)=refnum<vi> refnum, vi path=w275, options=w267, error in (no error)=w276) -> (vi reference=w269:refnum<vi>, error out=w270:errorcluster)  [unwired: 2 in]
        n119 = call-by-ref "Start Asynchronous Call"(reference=w269, error in=w270, "inIcon"=T24."Error", "inTitle"="ERROR", "inMessage"=w266) -> (reference out=w272:refnum<vi>, error out=w271:errorcluster)  [unwired: 6 in, 3 out]
        n120 = Close Reference(reference=w272, error in (no error)=w271) -> (error out=w273:errorcluster)
        n121 = call <vilib>:"Simple Error Handler.vi"("error in (no error)"=w273) -> ()  [unwired: 4 in, 5 out]
        n122 = Merge Errors(w282) -> (w281:errorcluster)
      }
      frame "Confirm Quit" {
        # "Confirm Quit - Message that can confirm whether or not the user wants to exit the application."
        n123 = call "NewDialog.vi"("inIcon"=T24."Information", "inTitle"="SHUTDOWN?", "inButton2Text"="Shutdown", "inButton1Text"="", "inMessage"="Are you sure you want to shutdown?") -> ("outButton2"=→"Shutdown?":bool)  [unwired: 4 in, 2 out]
        n124 = call-poly "Enqueue Message.vi"("Priority Message? (F)"=TRUE, "error in (no error)"=w300, "Message"="Exit", "Message Queue"=w296) -> ("error out"=w297:errorcluster)  [unwired: 6 in, 1 out]
        n125 = Merge Errors(w297) -> (w298:errorcluster)
      }
      frame "Exit" {
        # "Stop the VI"
        # "Release the message queue reference"
        # "Exit - Exit the application."
        n126 = Variant To Data(type=errorcluster {"status"=FALSE, "code"=0, "source"=""} ("error constant"), Variant=w305) -> (data=w306:errorcluster)  [unwired: 1 in, 1 out]
        n127 = call <vilib>:"Simple Error Handler.vi"("error in (no error)"=w306) -> ()  [unwired: 4 in, 5 out]
        n128 = Send Notification(notification=TRUE, notifier=w304) -> (error out=w302:errorcluster)  [unwired: 1 in, 1 out]
        n129 = call "Fire User Event - Stop.vi"("User Event - Stop"=w310) -> ("error out"=w309:errorcluster)  [unwired: 10 in]
        n130 = Release Queue(queue=w315, error in (no error)=w308) -> (error out=w312:errorcluster)  [unwired: 1 in, 2 out]
        n131 = Merge Errors(w302, w309, w312) -> (w311:errorcluster)
      }
      frame Default {
        # "'Default' case only runs if there is a message that isn't defined in any of the other cases.  Output a programming error."
        n132 = xnode "Error Ring"("parameter 0"=w317) -> ("error out"=w318:errorcluster)
      }
    }
    n133 = call "Error Handler - Message Handling Loop.vi"("error in (no error)"=w48, "Message Queue"=w50) -> ("dup error in"=w49:errorcluster)  [unwired: 8 in, 1 out]
  }
  n134 = while {
    tunnel: w29 -> [w334]
    shift-right: [w332] -> w35
    shift-left: w32 -> [w333]
    tunnel: [w328] -> w33
    stop <- w330 stop-if-true
    # "Event Handling Loop"
    n135 = event shown="[2] \"Shutdown\": Value Change" {
      selector: w333 -> [_ _ _ _ _ _ _ _ _ _ _ _ _ _ _ _ _ _]
      dyn-events: [_ _ _ _ _ _ _ _ _ _ _ _ _ _ _ _ _ _] -> w332
      timeout: 500 -> [_ _ _ _ _ _ _ _ _ _ _ _ _ _ _ _ _ _]
      tunnel: [_ _ _ _ _ _ _ _ _ _ _ _ _ _ _ _ _ TRUE ("Discard?")] -> w330
      tunnel: w334 -> [w339 w343 w348 w352 w356 w360 w364 w369 w374 w379 w383 w388 w390 w411 w421 w430 w439 w441]
      tunnel: [w338 _ w347 w351 w355 w359 w363 w368 w373 w380 _ w386 w391 w412 _ _ _ _] -> w331
      tunnel: [w337 w343 w346 w350 w354 w358 w362 w367 w372 w379 w383 w387 w390 w411 w421 w430 w439 w441] -> w329
      event Panel Close? {
        n136 = event-data() -> ()  [unwired: 1 in, 1 out]
        n137 = call-poly "Enqueue Message.vi"("Priority Message? (F)"=TRUE, "Message"="Confirm Quit", "Message Queue"=w339) -> ("error out"=w338:errorcluster, "dup Message Queue"=w337:refnum<queue>)  [unwired: 7 in]
        n138 = event-data("Discard?"=TRUE) -> ()  [unwired: 1 in, 1 out]
      }
      event Timeout {
        n139 = event-data() -> ()  [unwired: 1 in, 1 out]
        n140 = Format Date/Time String(time format string (%c)="%d %b %Y | %I:%M:%S %p") -> (date/time string=→"Date-Time":string)  [unwired: 2 in]
      }
      event "Shutdown": Value Change {
        n141 = event-data() -> ()  [unwired: 1 in, 1 out]
        n142 = call-poly "Enqueue Message.vi"("Priority Message? (F)"=TRUE, "Message"="Confirm Quit", "Message Queue"=w348) -> ("error out"=w347:errorcluster, "dup Message Queue"=w346:refnum<queue>)  [unwired: 7 in]
      }
      event "Home Para", "Home Manual": Value Change {
        n143 = event-data() -> ()  [unwired: 1 in, 1 out]
        n144 = call-poly "Enqueue Message.vi"("Message"="Initialize", "Message Queue"=w352) -> ("error out"=w351:errorcluster, "dup Message Queue"=w350:refnum<queue>)  [unwired: 8 in]
      }
      event "Back Stats", "Back IO": Value Change {
        n145 = event-data() -> ()  [unwired: 1 in, 1 out]
        n146 = call-poly "Enqueue Message.vi"("Message"="Autocycle Back", "Message Queue"=w356) -> ("error out"=w355:errorcluster, "dup Message Queue"=w354:refnum<queue>)  [unwired: 8 in]
      }
      event "Stats": Value Change {
        n147 = event-data() -> ()  [unwired: 1 in, 1 out]
        n148 = call-poly "Enqueue Message.vi"("Message"="Autocycle Stats", "Message Queue"=w360) -> ("error out"=w359:errorcluster, "dup Message Queue"=w358:refnum<queue>)  [unwired: 8 in]
      }
      event "All IO": Value Change {
        n149 = event-data() -> ()  [unwired: 1 in, 1 out]
        n150 = call-poly "Enqueue Message.vi"("Message"="Autocycle IO", "Message Queue"=w364) -> ("error out"=w363:errorcluster, "dup Message Queue"=w362:refnum<queue>)  [unwired: 8 in]
      }
      event "Home AC": Value Change {
        n151 = event-data() -> ()  [unwired: 1 in, 1 out]
        n152 = call-poly "Enqueue Message.vi"("Message"="Initialize", "Message Queue"=w369) -> ("error out"=w368:errorcluster, "dup Message Queue"=w367:refnum<queue>)  [unwired: 8 in]
        n153 = call "Write NS (HMI).vi"("Message"="Exit Autocycle") -> ()  [unwired: 10 in, 1 out]
      }
      event "Maintenance", "Parameters", "Manual": Value Change {
        n154 = event-data() -> ("CtlRef"=w371:refnum<vi>)  [unwired: 1 in]
        n155 = property class="Bool"(reference=w371) -> ("Label.Text"=w370:string)  [unwired: 1 in, 2 out]
        n156 = call-poly "Enqueue Message.vi"("Message"=w370, "Message Queue"=w374) -> ("error out"=w373:errorcluster, "dup Message Queue"=w372:refnum<queue>)  [unwired: 8 in]
      }
      event "Enable Insertion?", "Enable Cutting?", "Enable TF?", "Enable PF?", "Enable Index?", "Enable Measure?", "Enable Reject?", "Enable Agitate?", "Enable BF?": Value Change {
        n157 = event-data() -> ("CtlRef"=w381:refnum<vi>, "NewVal"=w375:bool)  [unwired: 1 in, 1 out]
        n158 = property class="Bool (strict)"(reference=w381) -> ("Label.Text"=w378:string)  [unwired: 1 in, 2 out]
        n159 = Concatenate Strings("GV:" ("string"), w378) -> (w376:string)
        n160 = call "Write NS (HMI).vi"("Message Data"=w375, "Message"=w376) -> ("error out"=w380:errorcluster)  [unwired: 9 in]
      }
      event "Reset MCount": Value Change {
        n161 = event-data() -> ()  [unwired: 1 in, 6 out]
        n162 = call-poly "Enqueue Message.vi"("Message"="Reset Manual Count", "Message Queue"=w383) -> ()  [unwired: 8 in, 2 out]
      }
      event "Run Manual": Value Change {
        n163 = event-data() -> ("CtlRef"=w385:refnum<vi>)  [unwired: 1 in, 2 out]
        n164 = property class="Bool"(reference=w385) -> ("Label.Text"=w384:string)  [unwired: 1 in, 2 out]
        n165 = call-poly "Enqueue Message.vi"("Message"=w384, "Message Queue"=w388) -> ("error out"=w386:errorcluster, "dup Message Queue"=w387:refnum<queue>)  [unwired: 8 in]
      }
      event "Toggle Motor": Value Change {
        n166 = event-data() -> ()  [unwired: 1 in, 3 out]
        n167 = call "Write NS (HMI).vi"("Message"="Toggle Motor") -> ("error out"=w391:errorcluster)  [unwired: 10 in]
      }
      event "Save Para": Value Change {
        n168 = event-data() -> ()  [unwired: 1 in, 3 out]
        n169 = Cluster To Array(cluster="Agitator Para") -> (array=w406:u32[])
        n170 = Cluster To Array(cluster="Tube Feeder Para") -> (array=w404:u32[])
        n171 = Cluster To Array(cluster="Insertion Para") -> (array=w402:u32[])
        n172 = Cluster To Array(cluster="Cutting Para") -> (array=w400:u32[])
        n173 = Cluster To Array(cluster="PF Para") -> (array=w398:u32[])
        n174 = Cluster To Array(cluster="Meas. Para") -> (array=w396:dbl[])
        n175 = Cluster To Array(cluster="Reject Para") -> (array=w394:u32[])
        n176 = Cluster To Array(cluster="BF Para") -> (array=w392:u32[])
        n177 = Bundle By Name(cluster=T7 {"Agitator Delays"=[1000], "TF Delays"=[1000], "Insertion Delays"=[1000], "Cutting Delays"=[1000], "PF Delays"=[1000], "Measur. Delays"=[1000.0], "Reject Delays"=[1000], "BF Delays"=[1000]} ("Auto Para"), "Agitator Delays"=w406, "TF Delays"=w404, "Insertion Delays"=w402, "Cutting Delays"=w400, "PF Delays"=w398, "Measur. Delays"=w396, "Reject Delays"=w394, "BF Delays"=w392) -> (w408:T7)
        n178 = call "Write NS (HMI).vi"("Message Data"=w408, "Message"="Save Para") -> ("error out"=w412:errorcluster)  [unwired: 9 in]
      }
      event "Insertion Para.Delay 1", "Insertion Para.Delay 2", "Agitator Para.Delay", "Agitator Para.Timeout", "Cutting Para.Delay", "Cutting Para.Delay 2", "Cutting Para.Delay 3", "Tube Feeder Para.Delay", "Tube Feeder Para.Delay 2", "Tube Feeder Para.Max Attempts", "PF Para.Delay", "PF Para.Timeout", "Reject Para.Delay", "BF Para.Delay 1", "BF Para.Delay 2": Mouse Up {
        n179 = event-data() -> ("CtlRef"=w413:refnum<vi>)  [unwired: 1 in, 4 out]
        n180 = property class="DigNum (strict)"(reference=w413) -> (reference out=w416:refnum<vi>, "Value"=w417:u32)  [unwired: 1 in, 1 out]
        n181 = Number To Fractional String(number=w417, precision (6)=0.0 ("width (-)")) -> (F-format string=w415:string)  [unwired: 2 in]
        n182 = call <userlib>:"HMI Pop Up Num KP v1.1.vi"("String In"=w415) -> ("String Out"=w414:string)  [unwired: 9 in, 1 out]
        n183 = Fract/Exp String To Number(string=w414, default (0 dbl)=0.0 ("default (0 I32)")) -> (number=w419:dbl)  [unwired: 2 in, 1 out]
        n184 = property class="DigNum (strict)"(reference=w416, "Value"=w419) -> ()  [unwired: 1 in, 2 out]
      }
      event "Meas. Para.Delay": Mouse Up {
        n185 = event-data() -> ("CtlRef"=w422:refnum<vi>)  [unwired: 1 in, 4 out]
        n186 = property class="DigNum (strict)"(reference=w422) -> (reference out=w425:refnum<vi>, "Value"=w426:dbl)  [unwired: 1 in, 1 out]
        n187 = Number To Fractional String(number=w426, precision (6)=0.0 ("width (-)")) -> (F-format string=w424:string)  [unwired: 2 in]
        n188 = call <userlib>:"HMI Pop Up Num KP v1.1.vi"("String In"=w424) -> ("String Out"=w423:string)  [unwired: 9 in, 1 out]
        n189 = Fract/Exp String To Number(string=w423, default (0 dbl)=0.0 ("default (0 I32)")) -> (number=w428:dbl)  [unwired: 2 in, 1 out]
        n190 = property class="DigNum (strict)"(reference=w425, "Value"=w428) -> ()  [unwired: 1 in, 2 out]
      }
      event "Meas. Para.Mean Length", "Meas. Para.Tolerance": Mouse Up {
        n191 = event-data() -> ("CtlRef"=w431:refnum<vi>)  [unwired: 1 in, 4 out]
        n192 = property class="DigNum (strict)"(reference=w431) -> (reference out=w434:refnum<vi>, "Value"=w435:dbl)  [unwired: 1 in, 1 out]
        n193 = Number To Fractional String(number=w435, precision (6)=1.0 ("width (-)")) -> (F-format string=w433:string)  [unwired: 2 in]
        n194 = call <userlib>:"HMI Pop Up Num KP v1.1.vi"("String In"=w433) -> ("String Out"=w432:string)  [unwired: 9 in, 1 out]
        n195 = Fract/Exp String To Number(string=w432, default (0 dbl)=0.0 ("default (0 I32)")) -> (number=w437:dbl)  [unwired: 2 in, 1 out]
        n196 = property class="DigNum (strict)"(reference=w434, "Value"=w437) -> ()  [unwired: 1 in, 2 out]
      }
      event User Event {
        # "The Message Handling Loop processed an \"Exit\" message, which fired this event to stop the Event Handling Loop."
        n197 = event-data() -> ()  [unwired: 1 in, 1 out]
      }
    }
    n198 = call "Error Handler - Event Handling Loop.vi"("error in (no error)"=w331, "Message Queue"=w329) -> ("dup error in"=w328:errorcluster)  [unwired: 8 in, 1 out]
  }
  n199 = call "HMI-cRIO Connection Manager.vi"("error in"=w1, "notifier in"=w2, "Queue in"=w29) -> ("error out"=w23:errorcluster, "Notifier out"=w24:refnum<notifier>)  [unwired: 7 in]
  n200 = Unregister For Events(event registration refnum=w35, error in=w33) -> (error out=w36:errorcluster)
  n201 = Merge Errors(w36, w38, w23) -> (w37:errorcluster)
  n202 = call "Destroy User Event - Stop.vi"("error in (no error)"=w37, "User Event - Stop"=w31) -> ("error out"=w26:errorcluster)  [unwired: 9 in]
  n203 = Release Notifier(notifier=w24, error in (no error)=w26) -> (error out=w25:errorcluster)  [unwired: 1 in, 2 out]
  n204 = disable-structure shown="RUN_TIME_ENGINE==True" {
    disable-tunnel: w25 -> [_ _]
    frame condition #0 (active) {
    }
    frame condition #1 {
      # "Call Quit LabVIEW if running as a built application."
      n205 = Quit LabVIEW() -> ()  [unwired: 1 in]
    }
  }
